vi "PositionTracer.vi"() -> ()   [LabVIEW 2012]
panel:
  in  "delay (s)":dbl=-0.9
  out "Y out chart":dbl(graph)
  out "X out chart":dbl(graph)
  out "Y out":dbl
  out "X out":dbl
  out "logical OR":bool
  out "empty?":bool
  out "Image":T1(plugin-control)
  in  "Tracking file":path=path "C:/Users/Ludovico/Lavoro/Experiments/Autofocus/vermi/track3.txt"
  in  "Pixel size":sgl=1.6
  in  "Settings":T2={"Objects"=1, "Threshold"=90, "Reject Border"=FALSE, "Fill Holes"=FALSE, "Min Object Size"=TRUE, "Min Size"=3000, "Max Object Size"=TRUE, "Max Size"=100000, "Show Search Area"=FALSE, "Show Center"=TRUE, "Show Bounding Box"=TRUE} {"Objects" items=["Bright Objects", "Dark Objects"]; "Threshold" min=1 max=999999999 step=1; "Max Size" min=1 max=999999999 step=1; "Min Size" min=1 max=999999999 step=1}
  in  "Interframe time (s)":dbl=0.1
  in  "Image file pattern":string="*tif*"
  in  "Positions file":path=path "C:/Users/Ludovico/Lavoro/Experiments/Autofocus/vermi/CONFSTAGELOG/2016_12_16_10_06.txt"
  in  "Input images folder":path=path "C:/Users/Ludovico/Lavoro/Experiments/Autofocus/vermi/161216_1c_reduced"
  out "error out":errorcluster
  in  "error in (no error)":errorcluster
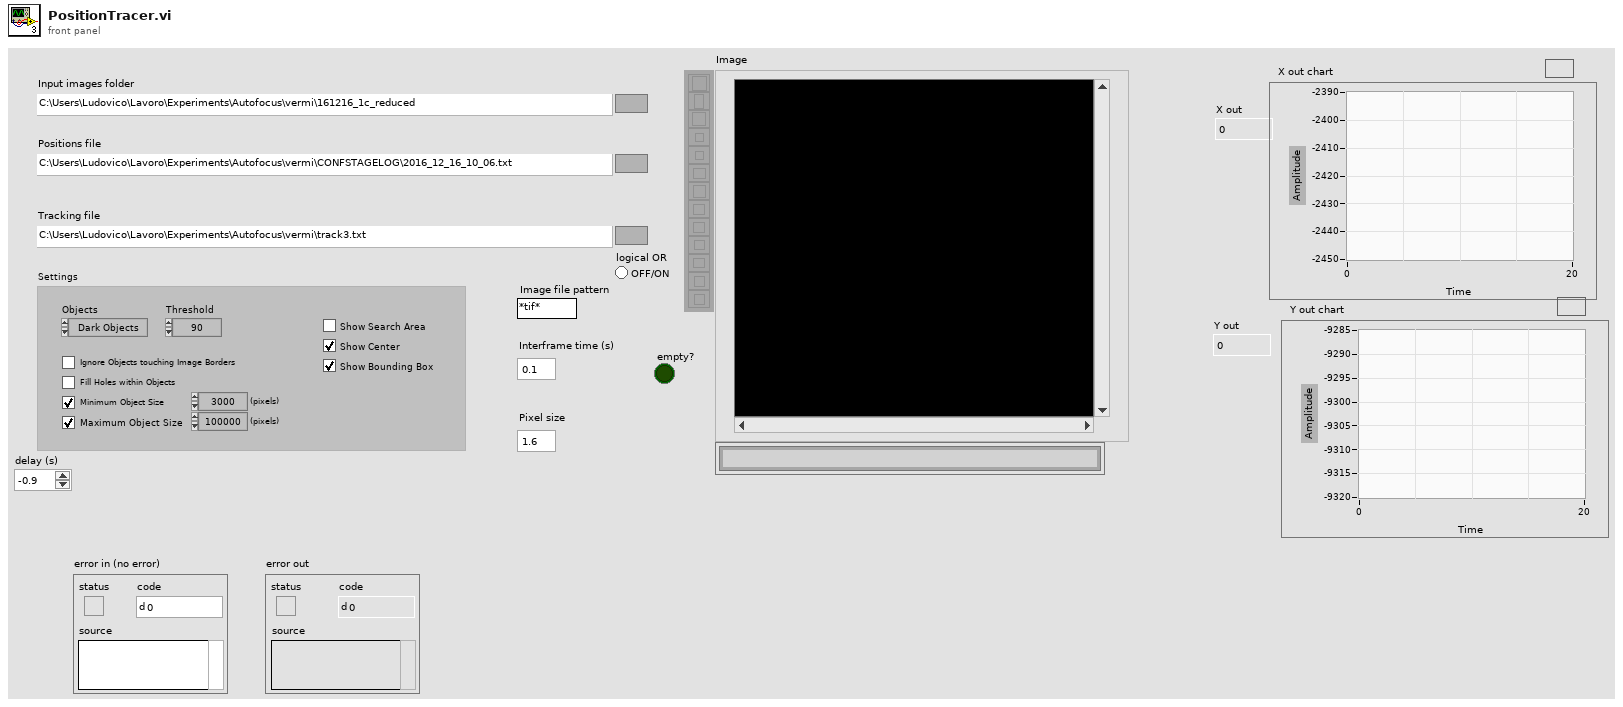
[diagram p1: front panel]
types:
  T1 = typedef "IMAQ Image.ctl" = refnum<image>
  T2 = cluster{"Objects":u16, "Threshold":i32, "Reject Border":bool, "Fill Holes":bool, "Min Object Size":bool, "Min Size":i32, "Max Object Size":bool, "Max Size":i32, "Show Search Area":bool, "Show Center":bool, "Show Bounding Box":bool}
  T3 = cluster{"X":dbl[], "Y":dbl[], "Focus":dbl[], "Time array":dbl[]}
  T4 = cluster{"Object Center":cluster{"X":sgl, "Y":sgl}, "Bounding Box":cluster{"X Left":i32, "Y Top":i32, "X Right":i32, "Y Bottom":i32}, "Area":sgl, "Orientation":sgl, "Aspect Ratio":sgl, "Nb Holes":i32}[]
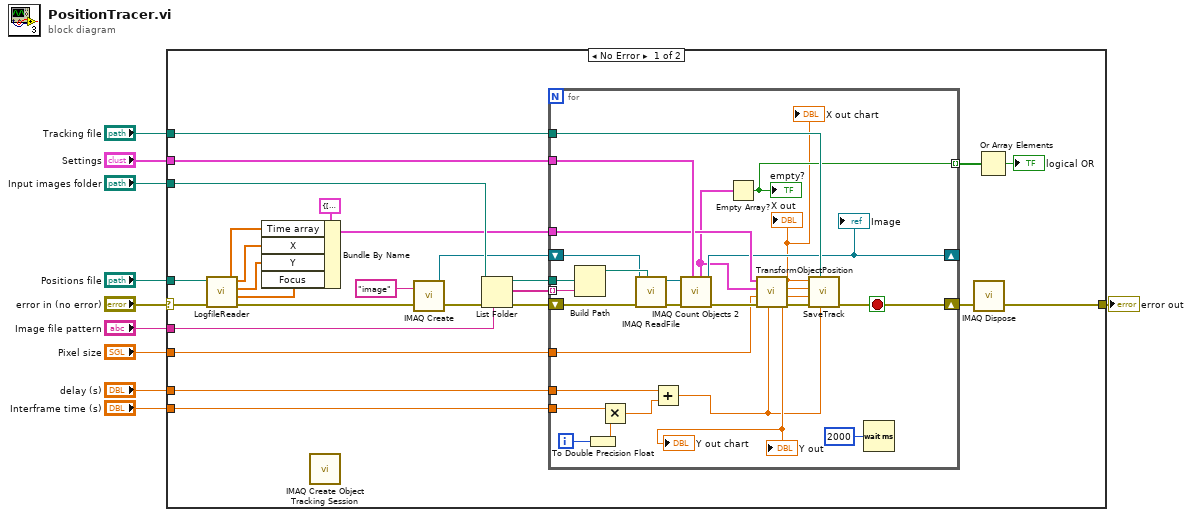
[diagram p0: block diagram]
diagram:
  n1 = case shown="No Error" "error in (no error)" {
    selector: "error in (no error)" -> [w36 w64]
    tunnel: "Positions file" -> [w32 _]
    tunnel: "Input images folder" -> [w31 _]
    tunnel: "Image file pattern" -> [w30 _]
    tunnel: "Interframe time (s)" -> [w18 _]
    tunnel: "Settings" -> [w25 _]
    tunnel: "Pixel size" -> [w17 _]
    tunnel: "Tracking file" -> [w16 _]
    tunnel: [w14 w64] -> w2
    tunnel: "delay (s)" -> [w11 _]
    frame No Error {
      n2 = call "LogfileReader.vi"("error in (no error)"=w36, "Positions file"=w32) -> ("error out"=w34:errorcluster, "Focus"=w20:dbl[], "Y"=w21:dbl[], "X"=w22:dbl[], "Time"=w23:dbl[])  [unwired: 5 in]
      n3 = Bundle By Name(cluster=T3 {"X"=[], "Y"=[], "Focus"=[], "Time array"=[]} ("Spacetime cluster"), "Time array"=w23, "X"=w22, "Y"=w21, "Focus"=w20) -> (w19:T3)
      n4 = call "IMAQ Create Object Tracking Session"() -> ()  [unwired: 10 in, 2 out]
      n5 = call "IMAQ Create"("Image Name"="image", "error in (no error)"=w34) -> ("New Image"=w26:T1, "error out"=w33:errorcluster)  [unwired: 3 in]
      n6 = List Folder(path=w31, pattern=w30, error in=w33) -> (path out=w27:path, filenames=w28:string[], error out=w29:errorcluster)  [unwired: 1 in, 1 out]
      n7 = for {
        tunnel: w28 -> [w62] mode=indexing
        tunnel: w27 -> [w61]
        shift-right: [w45] -> w15
        shift-left: w29 -> [w63]
        shift-right: [w46] -> _
        shift-left: w26 -> [w59]
        tunnel: w25 -> [w56]
        tunnel: w19 -> [w54]
        tunnel: w18 -> [w51]
        tunnel: w17 -> [w50]
        tunnel: w16 -> [w47]
        tunnel: [w42] -> w13 mode=indexing
        tunnel: w11 -> [w37]
        i -> [w53]
        stop <- w45 stop-if-true
        n8 = Build Path(base path=w61, name or relative path=w62) -> (appended path=w60:path)
        n9 = To Double Precision Float(number=w53) -> (double precision float=w52:dbl)
        n10 = Multiply(x=w51, y=w52) -> (x*y=w39:dbl)
        n11 = call "IMAQ ReadFile"("File Path"=w60, "error in (no error)"=w63, "Image"=w59) -> ("error out"=w57:errorcluster, "Image Out"=w58:T1)  [unwired: 4 in, 3 out]
        n12 = Add(x=w37, y=w39) -> (x+y=w38:dbl)
        n13 = call "IMAQ Count Objects 2"("Settings"=w56, "error in (no error)"=w57, "Image"=w58) -> ("error out"=w55:errorcluster, "Image Out"=w46:T1, "Objects"=w43:T4)  [unwired: 4 in, 2 out]
        "Image" <- w46
        n14 = Empty Array?(array=w43) -> (empty?=w42:bool)
        "empty?" <- w42
        n15 = call "TransformObjectPosition.vi"("Image time"=w38, "error in (no error)"=w55, "Pixel size"=w50, "Objects"=w43, "Spacetime cluster"=w54) -> ("error out"=w49:errorcluster, "Focus out"=w48:dbl, "Y out"=w40:dbl, "X out"=w41:dbl)  [unwired: 3 in]
        "X out" <- w41
        "Y out" <- w40
        "X out chart" <- w41
        "Y out chart" <- w40
        n16 = call "SaveTrack.vi"("Time"=w38, "Track file"=w47, "error in (no error)"=w49, "Focus"=w48, "Y"=w40, "X"=w41) -> ("error out"=w45:errorcluster)  [unwired: 5 in]
        n17 = Wait (ms)(milliseconds to wait=u32 2000) -> ()  [unwired: 1 out]
      }
      n18 = call "IMAQ Dispose"("error in (no error)"=w15) -> ("error out"=w14:errorcluster)  [unwired: 5 in]
      n19 = Or Array Elements(Boolean array=w13) -> (logical OR=→"logical OR":bool)
    }
    frame Error {
    }
  }
  "error out" <- w2
